vi "Query Arb Sequence Capabilities [SEQ] Core.vi"(8 "error in (no error)":errorcluster, 11 "IVI_Fgen in":refnum<class "IVI_Fgen.lvclass">) -> (0 "error out":errorcluster, 1 "min sequence length":i32, 2 "max number of sequences":i32, 3 "IVI_Fgen out":refnum<class "IVI_Fgen.lvclass">, 4 "max sequence length":i32, 6 "max loop count":i32)   [LabVIEW 2013, in "IVI_Fgen.lvlib" / "IVI_Fgen.lvclass"]
doc: "This VI returns the properties of the function generator that are related to creating arbitrary sequences. These properties are the maximum number of sequences, minimum sequence length, maximum sequence length, and maximum loop count.\n\nNotes:\n\n(1) This VI is part of the IviFgenArbSeq [SEQ] extension group."
uses:
  IVI_Fgen.lvclass
  IVI_Fgen.lvclass/IVI_Fgen.ctl
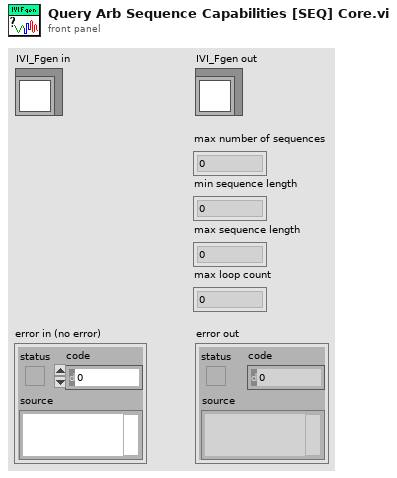
[diagram p1: front panel]
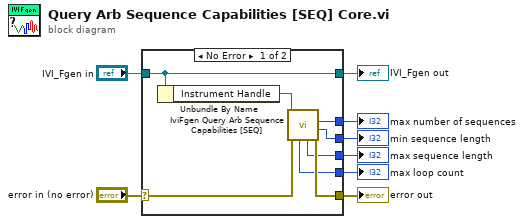
[diagram p0: block diagram]
diagram:
  n1 = case shown="No Error" "error in (no error)" {
    selector: "error in (no error)" -> [w14 w18]
    tunnel: [w13 w18] -> w7
    tunnel: [w16 w17] -> w5
    tunnel: "IVI_Fgen in" -> [w16 w17]
    tunnel: [w12 _] -> w4
    tunnel: [w11 _] -> w3
    tunnel: [w10 _] -> w2
    tunnel: [w9 _] -> w1
    frame No Error {
      n2 = Unbundle By Name(w16) -> ("Instrument Handle"=w15:refnum<k15>)
      n3 = call <vilib>:"IviFgen Query Arb Sequence Capabilities [SEQ].vi"("error in (no error)"=w14, "instrument handle"=w15) -> ("error out"=w13:errorcluster, "min sequence length"=w11:i32, "max number of sequences"=w12:i32, "max sequence length"=w10:i32, "max loop count"=w9:i32)  [unwired: 4 in, 1 out]
    }
    frame Error {
    }
  }
  "error out" <- w7
  "IVI_Fgen out" <- w5
  "max number of sequences" <- w4
  "min sequence length" <- w3
  "max sequence length" <- w2
  "max loop count" <- w1
